vi "LV Path to C Path.vi"(8 "错误输入（无错误）":errorcluster, 11 "Dir Path":path) -> (0 "错误输出":errorcluster, 3 "C Path":string)   [LabVIEW 2012, in "FileSystem Watcher.lvlib"]
uses:
  FileSystem Watcher.lvlib
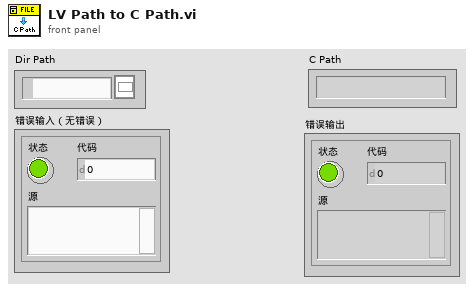
[diagram p1: front panel]
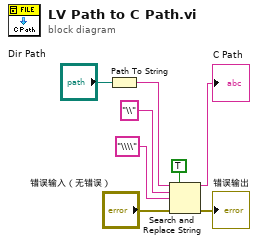
[diagram p0: block diagram]
diagram:
  n1 = Path To String(path="Dir Path") -> (string=w7:string)
  n2 = Search and Replace String(replace all?=TRUE ("替换全部？(F)"), input string=w7, search string="\\" ("搜索字符串"), replace string="\\\\" ("替换字符串(\"\")"), error in="错误输入（无错误）") -> (result string=→"C Path":string, error out=→"错误输出":errorcluster)  [unwired: 3 in, 2 out]
